vi "Write Device ID RF.vi"(8 "error in (no error)":errorcluster, 10 "Device ID RF":u8, 11 "NKT in":refnum<class "NKT_Extreme.lvclass">) -> (0 "error out":errorcluster, 3 "NKT out":refnum<class "NKT_Extreme.lvclass">)   [LabVIEW 2020, in "NKT_Extreme.lvclass"]
uses:
  <instrlib>/Classes/Laser/NKT/NKT_Extreme.lvclass
  <instrlib>/Classes/Laser/NKT/NKT_Extreme.lvclass/NKT_Extreme.ctl
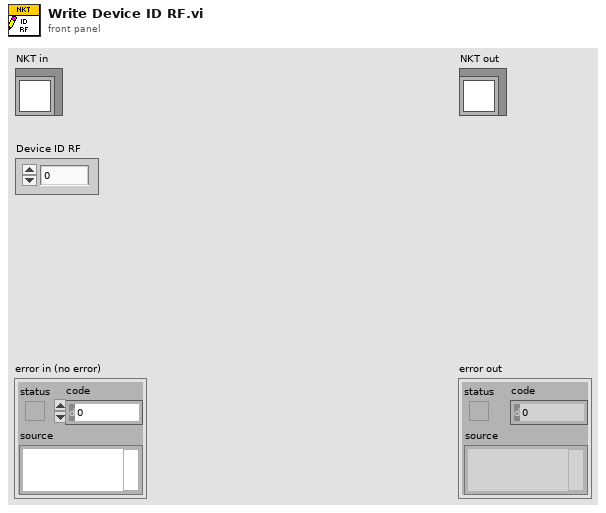
[diagram p1: front panel]
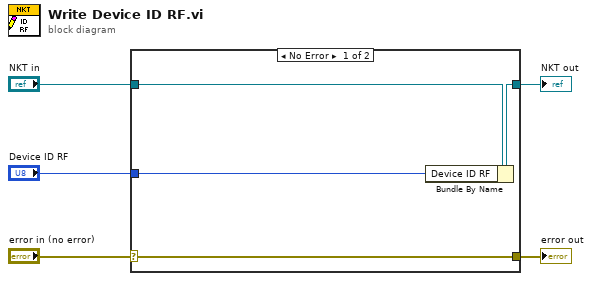
[diagram p0: block diagram]
diagram:
  n1 = case shown="No Error" "error in (no error)" {
    selector: "error in (no error)" -> [w9 w10]
    tunnel: [w9 w10] -> w4
    tunnel: [w7 w11] -> w2
    tunnel: "NKT in" -> [w8 w11]
    tunnel: "Device ID RF" -> [w6 _]
    frame No Error {
      n2 = Bundle By Name(cluster=w8, "Device ID RF"=w6) -> (w7:refnum<class "NKT_Extreme.lvclass">)
    }
    frame Error {
    }
  }
  "error out" <- w4
  "NKT out" <- w2
